vi "Jog.vi"(8 "NewVal":dbl[](array[numeric]), 9 "Old Var":dbl[](array[numeric]), 10 "error in (no error)":errorcluster, 11 "reference":refnum<k24>) -> (2 "error out":errorcluster, 3 "reference out":refnum<k24>)   [LabVIEW 2017]
uses:
  C:/KMotion434/KMotion/Release/KMotion_dotNet.dll
panel:
  out "Value 2":dbl
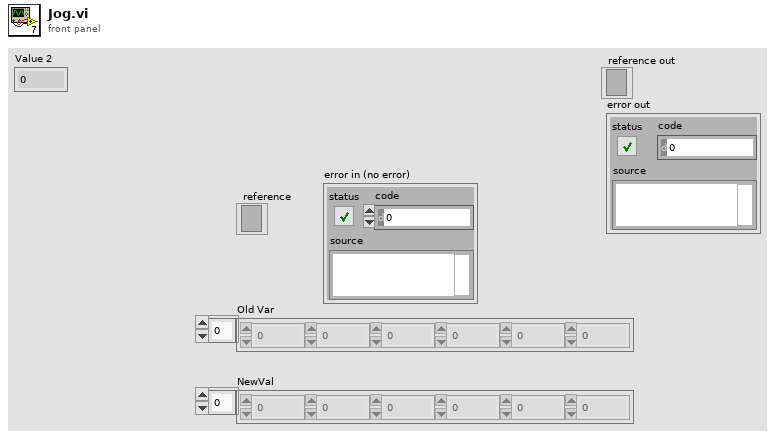
[diagram p1: front panel]
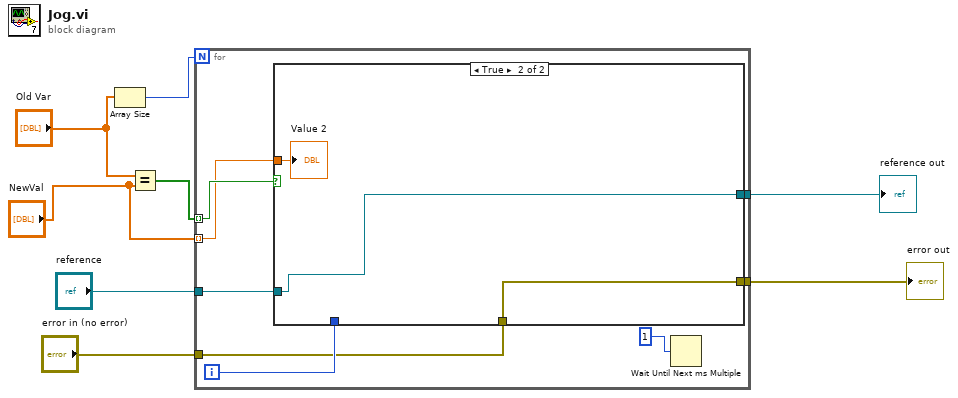
[diagram p0: block diagram]
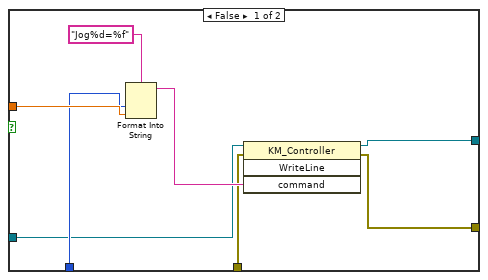
[diagram p2: hidden frame]
diagram:
  n1 = Array Size(array="Old Var") -> (size(s)=w7:i32)
  n2 = Equal?(x="Old Var", y="NewVal") -> (x = y?=w8:bool[])
  n3 = for {
    N: w7 -> [_]
    tunnel: w8 -> [w16] mode=indexing
    tunnel: "NewVal" -> [w15] mode=indexing
    tunnel: "error in (no error)" -> [w12]
    tunnel: "reference" -> [w11]
    tunnel: [w10] -> w2
    tunnel: [w9] -> w1
    i -> [w14]
    n4 = case shown="True" w16 {
      tunnel: w15 -> [w22 w27]
      tunnel: w14 -> [w21 _]
      tunnel: w12 -> [w20 w26]
      tunnel: w11 -> [w19 w25]
      tunnel: [w18 w26] -> w10
      tunnel: [w17 w25] -> w9
      frame False {
        n5 = Format Into String(format string="Jog%d=%f", w21, w22) -> (resulting string=w23:string)  [unwired: 2 in, 1 out]
        n6 = invoke class="KM_Controller" method="WriteLine"(reference=w19, error in=w20, "command"=w23) -> (reference out=w17:refnum<k24>, error out=w18:errorcluster)  [unwired: 1 in, 2 out]
      }
      frame True {
        "Value 2" <- w27
      }
    }
    n7 = Wait Until Next ms Multiple(millisecond multiple=u32 1) -> ()  [unwired: 1 out]
  }
  "error out" <- w2
  "reference out" <- w1
